vi "Math-Truncated Gaussian RNG.vi"(0 "samples":i32, 1 "reset":bool, 5 "Min":dbl, 7 "Max":dbl, 9 "mu":dbl, 11 "sigma":dbl, 12 "seed":i32=-1) -> (4 "Array":dbl[](array[numeric]))   [LabVIEW 2020]
uses:
  <vilib>/gmath/statdist.llb/Normal CDF.vi
  <vilib>/gmath/statdist.llb/Uniform Random.vi
  <vilib>/gmath/statdist.llb/Normal Inverse CDF.vi
  <vilib>/gmath/NI_Gmath.lvlib
  <vilib>/Analysis/NI_AALBase.lvlib
panel:
  out "Histogram":T1(graph)
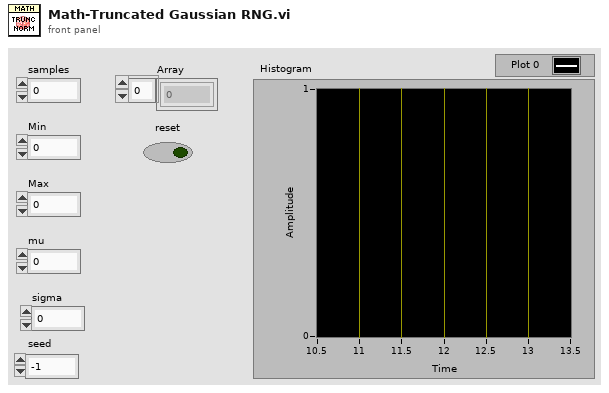
[diagram p1: front panel]
types:
  T1 = cluster{"X Values":dbl[], "Histogram: h(x)":i32[]}
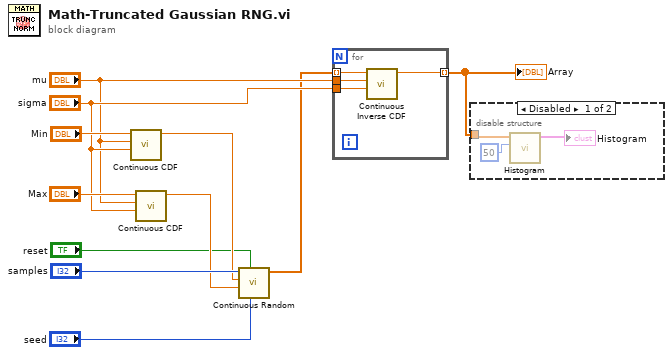
[diagram p0: block diagram]
diagram:
  n1 = call-poly <vilib>:"Continuous CDF.vi"("std"="sigma", "mean"="mu", "x"="Min") -> ("cdf(x)"=w8:dbl)  [unwired: 7 in, 1 out]
  n2 = call-poly <vilib>:"Continuous CDF.vi"("std"="sigma", "mean"="mu", "x"="Max") -> ("cdf(x)"=w4:dbl)  [unwired: 7 in, 1 out]
  n3 = call-poly <vilib>:"Continuous Random.vi"("seed"="seed", "reset"="reset", "xmax"=w4, "xmin"=w8, "samples"="samples") -> ("uniform random data"=w3:dbl[])  [unwired: 5 in, 1 out]
  n4 = for {
    tunnel: "sigma" -> [w15]
    tunnel: "mu" -> [w14]
    tunnel: w3 -> [w13] mode=indexing
    tunnel: [w12] -> w2 mode=indexing
    n5 = call-poly <vilib>:"Continuous Inverse CDF.vi"("std"=w15, "mean"=w14, "cdf(x)"=w13) -> ("x"=w12:dbl)  [unwired: 7 in, 1 out]
  }
  "Array" <- w2
  n6 = disable-structure shown="Disabled" {
    disable-tunnel: w2 -> [w18 _]
    frame Disabled {
      n7 = call <vilib>:"Histogram.vi"("intervals"=50, "X"=w18) -> ("Histogram Graph"=→"Histogram":T1)  [unwired: 6 in, 3 out]
    }
    frame Enabled {
    }
  }
